vi "Build Monitor Engine Configuration.vi"(6 "log thresholds":T2 {"Segment Files By" items=["Time", "Size"]}, 7 "log file info":T1, 8 "error in":errorcluster, 9 "port properties":T3, 10 "board properties":T4 {"portConfig" items=["FDX_SINGLE", "FDX_REDUNDANT"]; "portSpeed" items=["FDX_100MBIT", "FDX_10MBIT", "FDX_AUTO_100MBIT", "FDX_AUTO_10MBIT", "FDX_AUTO_ERROR", "FDX_1000MBIT"]}, 11 "section ref in":T9=18446744073709551615 format="%.0x") -> (0 "error out":errorcluster, 2 "Monitor cluster out":T5={"channel #"=0, "channel handle"=0, "InstrumentHandle_board"=0, "InstrumentHandle_port"=0, "Queue ID"=0, "channel settings"={"Monitor Settings"={"DefaultCronoMode"=0, "GlbMonBufferSizeIn"=0}, "Rx Board"=0, "Rx Port"=0}, "current log file name"=path "", "monitor queue settings"={"TriggerPosition"=0, "CaptureMode"=0, "Strobe"=0, "MaxFileSize MB (1)"=1}, "Log File Directory"="", "Base name"="", "Timestamp"=FALSE, "log thresholds"={"segmentation threshold"=0.0, "DiskSpaceThPerc"=0.0, "checkDiskSpace"=FALSE, "segmentFiles"=FALSE, "Segment Files By"=0}} {"log thresholds"."Segment Files By" items=["Time", "Size"]; "monitor queue settings"."Strobe" items=["FDX_MON_STROBE_DIS", "FDX_MON_STROBE_STOP", "FDX_MON_STROBE_START"]; "monitor queue settings"."CaptureMode" items=["FDX_MON_SINGLE ", "FDX_MON_CONTINUOUS", "FDX_MON_SELECTIVE", "FDX_MON_RECORDING", "FDX_MON_REROS", "FDX_MON_HMU"]; "channel settings"."Monitor Settings"."DefaultCronoMode" items=["FDX_RX_DEFAULT_ENA_CNT", "FDX_RX_DEFAULT_MON_ENA_ALL", "FDX_RX_DEFAULT_MON_ENA_GOOD"]}, 3 "section ref out":T9 format="%.0x")   [LabVIEW 2020, in "AIM ARINC 664 Scripting.lvlib"]
uses:
  AIM ARINC 664 Scripting.lvlib
  <vilib>/NI VeriStand/Custom Device API/Custom Device Item Ref.ctl
  Shared/hardware_channels_rx.ctl
  Shared/channel_settings_rx.ctl
  <instrlib>/AIM GmbH/_AIM 664/_controls/session_monitor_config.ctl
  Shared/monitor_queue_settings.ctl
  Shared/loggingThreshold_types.ctl
  Shared/board_setup.ctl
  Shared/port_setup.ctl
  Shared/session_rx_monitor.ctl
  <instrlib>/AIM GmbH/_AIM 664/AIM664LV.lvlib
  Import/AIM ARINC 664 Import.lvlib
  <vilib>/NI VeriStand/Custom Device API/Custom Device API.lvlib
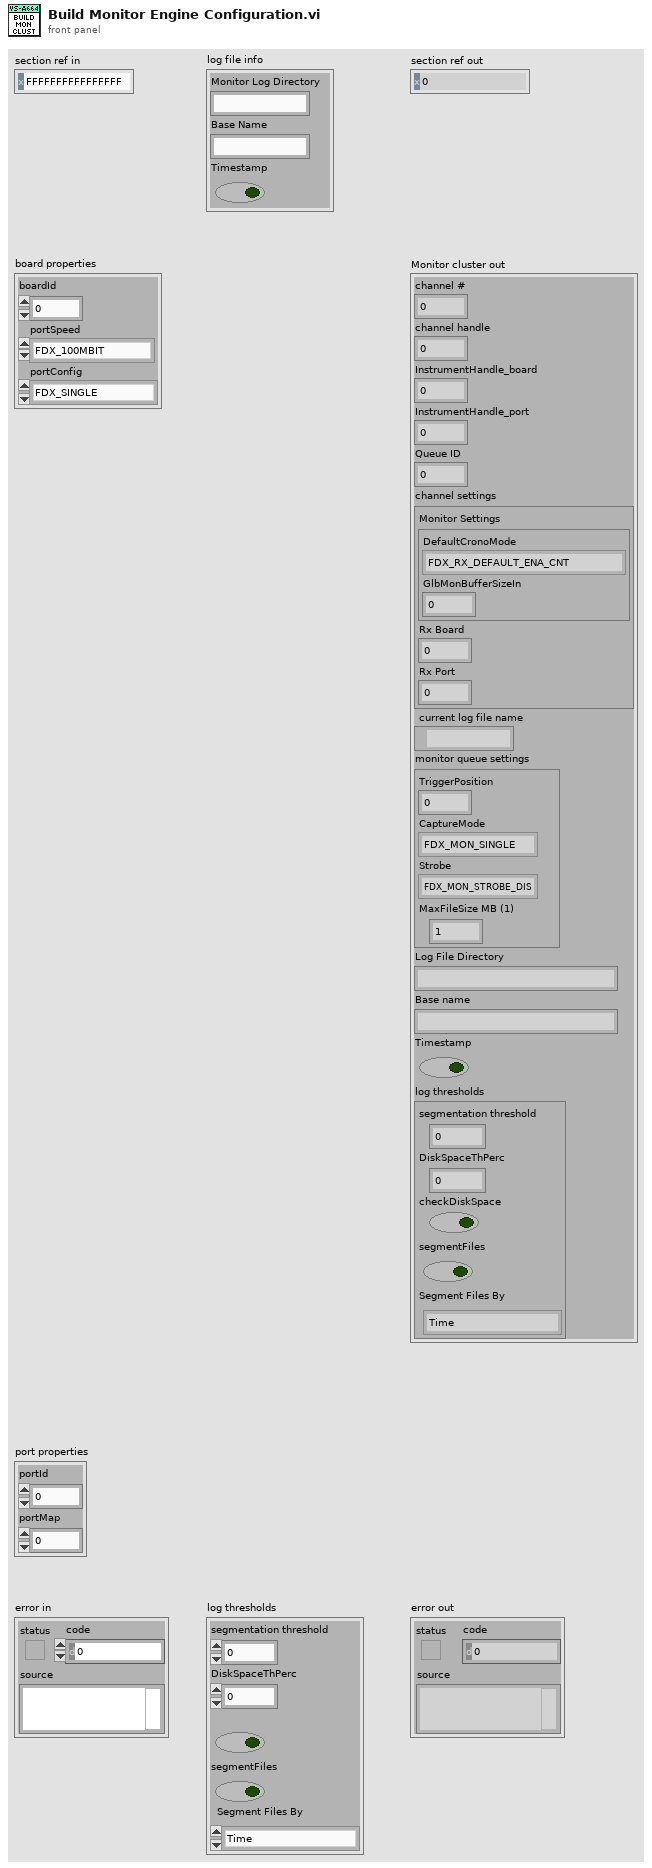
[diagram p1: front panel]
types:
  T1 = cluster{"Monitor Log Directory":string, "Base Name":string, "Timestamp":bool}
  T2 = typedef "loggingThreshold_types.ctl" = cluster{"segmentation threshold":dbl, "DiskSpaceThPerc":dbl, "checkDiskSpace":bool, "segmentFiles":bool, "Segment Files By":u16}
  T3 = typedef "AIM ARINC 664 Import.lvlib/port_setup.ctl" = cluster{"portId":u32, "portMap":u32}
  T4 = typedef "AIM ARINC 664 Import.lvlib/board_setup.ctl" = cluster{"boardId":u32, "portSpeed":u32, "portConfig":u32}
  T5 = typedef "hardware_channels_rx.ctl" = cluster{"channel #":u16, "channel handle":u64, "InstrumentHandle_board":u32, "InstrumentHandle_port":u32, "Queue ID":u32, "channel settings":T6, "current log file name":path, "monitor queue settings":T8, "Log File Directory":string, "Base name":string, "Timestamp":bool, "log thresholds":T2}
  T6 = typedef "channel_settings_rx.ctl" = cluster{"Monitor Settings":T7, "Rx Board":u32, "Rx Port":u32}
  T7 = typedef "AIM664LV.lvlib/session_monitor_config.ctl" = cluster{"DefaultCronoMode":u32, "GlbMonBufferSizeIn":u32}
  T8 = typedef "monitor_queue_settings.ctl" = cluster{"TriggerPosition":u32, "CaptureMode":u32, "Strobe":u32, "MaxFileSize MB (1)":u32}
  T9 = typedef "Custom Device API.lvlib/Custom Device Item Ref.ctl" = u64
  T10 = typedef "AIM ARINC 664 Import.lvlib/session_rx_monitor.ctl" = cluster{"DefaultCronoMode":u32, "GlbMonBufferSizeIn":u32, "CaptureMode":u32, "MaxFileSizeMB":u32, "Strobe":u32, "TriggerPosition":u32}
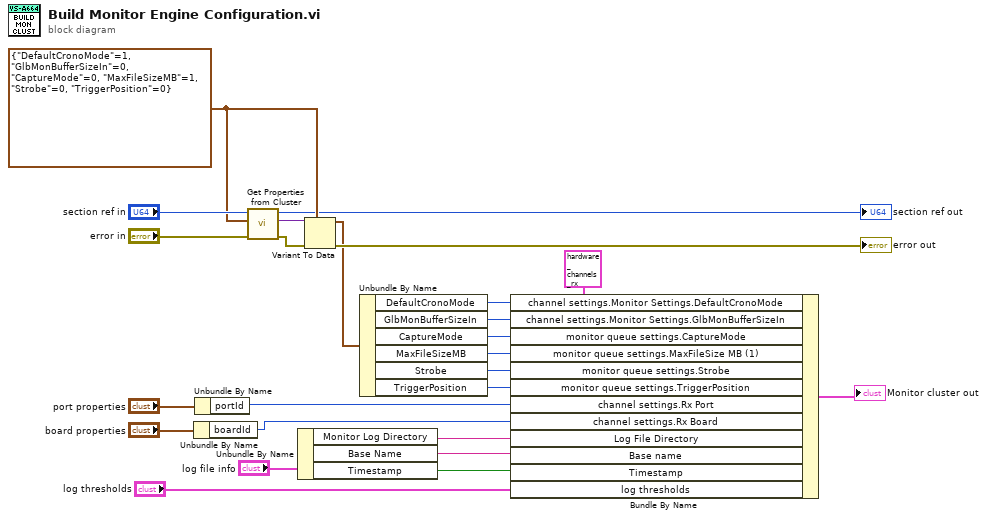
[diagram p0: block diagram]
diagram:
  w19 = T10 {"DefaultCronoMode"=1, "GlbMonBufferSizeIn"=0, "CaptureMode"=0, "MaxFileSizeMB"=1, "Strobe"=0, "TriggerPosition"=0} ("session_rx_monitor")
  n1 = Unbundle By Name("board properties") -> ("boardId"=w13:u32)
  n2 = Unbundle By Name("port properties") -> ("portId"=w14:u32)
  n3 = call "Get Properties from Cluster.vi"("error in"="error in", "Variant Cluster"=w19, "custom device ref in"="section ref in") -> ("error out"=w20:errorcluster, "data"=w21:variant, "custom device ref out"=→"section ref out":T9)  [unwired: 5 in, 1 out]
  n4 = Unbundle By Name("log file info") -> ("Monitor Log Directory"=w3:string, "Base Name"=w2:string, "Timestamp"=w1:bool)
  n5 = Variant To Data(error in=w20, type=w19, Variant=w21) -> (data=w12:T10, error out=→"error out":errorcluster)
  n6 = Unbundle By Name(w12) -> ("DefaultCronoMode"=w11:u32, "GlbMonBufferSizeIn"=w10:u32, "CaptureMode"=w9:u32, "MaxFileSizeMB"=w8:u32, "Strobe"=w7:u32, "TriggerPosition"=w6:u32)
  n7 = Bundle By Name(cluster=T5 {"channel #"=0, "channel handle"=0, "InstrumentHandle_board"=0, "InstrumentHandle_port"=0, "Queue ID"=0, "channel settings"={"Monitor Settings"={"DefaultCronoMode"=1, "GlbMonBufferSizeIn"=0}, "Rx Board"=0, "Rx Port"=1}, "current log file name"=path "", "monitor queue settings"={"TriggerPosition"=0, "CaptureMode"=1, "Strobe"=0, "MaxFileSize MB (1)"=1}, "Log File Directory"="", "Base name"="", "Timestamp"=FALSE, "log thresholds"={"segmentation threshold"=0.0, "DiskSpaceThPerc"=0.0, "checkDiskSpace"=FALSE, "segmentFiles"=FALSE, "Segment Files By"=0}} ("RX Parameters"), "channel settings.Monitor Settings.DefaultCronoMode"=w11, "channel settings.Monitor Settings.GlbMonBufferSizeIn"=w10, "monitor queue settings.CaptureMode"=w9, "monitor queue settings.MaxFileSize MB (1)"=w8, "monitor queue settings.Strobe"=w7, "monitor queue settings.TriggerPosition"=w6, "channel settings.Rx Port"=w14, "channel settings.Rx Board"=w13, "Log File Directory"=w3, "Base name"=w2, "Timestamp"=w1, "log thresholds"="log thresholds") -> (→"Monitor cluster out":T5)
